vi "Simple App.vi"() -> ()   [LabVIEW 2014, in "SR3XXX HVPS.lvclass"]
uses:
  SR3XXX HVPS.lvclass
  reusable/Session APIs/Serial/Serial Session.lvclass
  reusable/Session APIs/Serial/Typedefs/Session Handle.ctl
panel:
  out "STB":bool[](array[boolean])
  out "ESB":bool[](array[boolean])
  in  "Power":bool
  out "voltage":dbl
  in  "Voltage Lim":dbl
  in  "Voltage SP":dbl
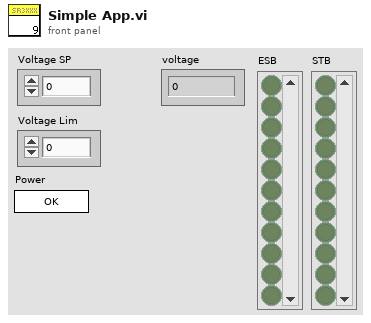
[diagram p1: front panel]
types:
  T1 = typedef "Serial Session.lvclass/Session Handle.ctl" = refnum<data-value>
  T2 = typedef "Session - Root.lvclass/Session Handle.ctl" = refnum<data-value>
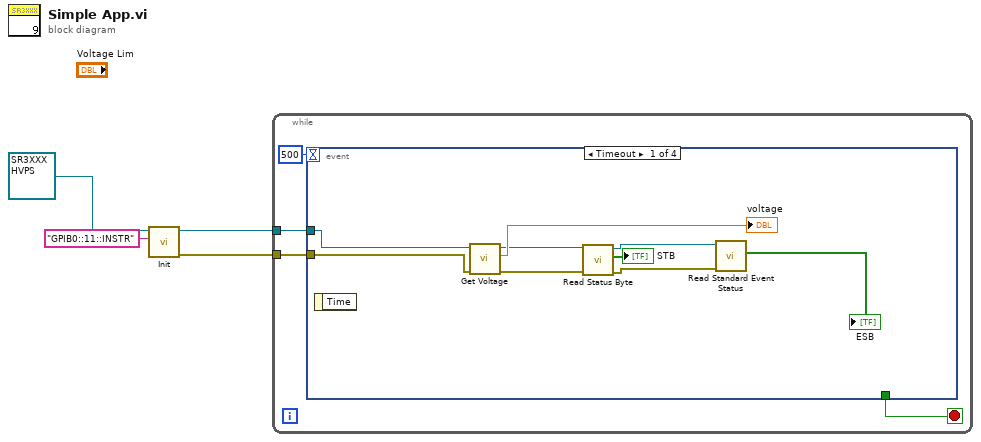
[diagram p0: block diagram]
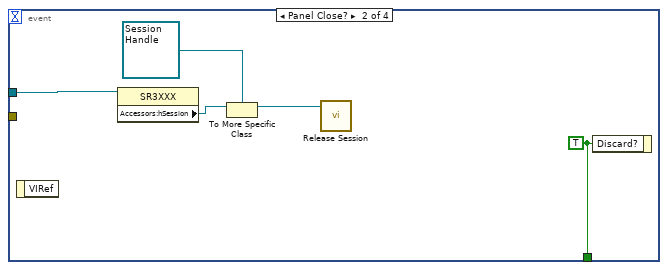
[diagram p2: hidden frame]
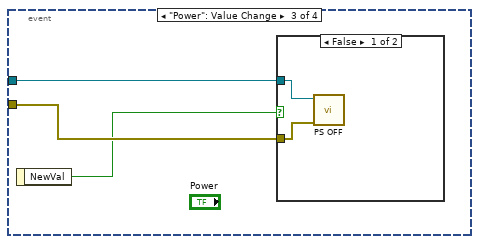
[diagram p3: hidden frame]
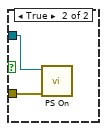
[diagram p4: hidden frame]
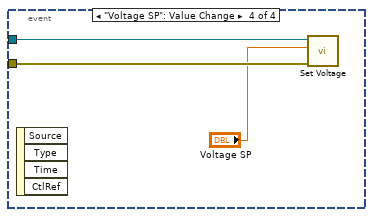
[diagram p5: hidden frame]
diagram:
  n1 = call-dynamic "Init.vi"("Session"="GPIB0::11::INSTR", "SR3XXX HVPS in"=refnum<class "SR3XXX HVPS.lvclass"> refnum) -> ("error out"=w1:errorcluster, "SR3XXX HVPS out"=w2:refnum<class "SR3XXX HVPS.lvclass">)  [unwired: 8 in]
  n2 = while {
    tunnel: w2 -> [w7]
    tunnel: w1 -> [w6]
    stop <- w8 stop-if-true
    n3 = event shown="[0] Timeout" {
      selector: _ -> [_ _ _ _]
      dyn-events: _ -> [_ _ _ _]
      timeout: 500 -> [_ _ _ _]
      tunnel: [_ w22 _ _] -> w8
      tunnel: w7 -> [w17 w21 w25 w32]
      tunnel: w6 -> [w16 _ w24 w31]
      event Timeout {
        n4 = event-data() -> ()  [unwired: 1 in, 1 out]
        n5 = call-dynamic "Get Voltage.vi"("error in (no error)"=w16, "SR3XXX HVPS in"=w17) -> ("error out"=w13:errorcluster, "V"=→"voltage":dbl, "SR3XXX HVPS out"=w14:refnum<class "SR3XXX HVPS.lvclass">)  [unwired: 7 in]
        n6 = call-dynamic "Read Status Byte.vi"("error in (no error)"=w13, "SR3XXX HVPS in"=w14) -> ("error out"=w11:errorcluster, "Byte"=→"STB":bool[], "SR3XXX HVPS out"=w12:refnum<class "SR3XXX HVPS.lvclass">)  [unwired: 7 in]
        n7 = call-dynamic "Read Standard Event Status.vi"("error in (no error)"=w11, "SR3XXX HVPS in"=w12) -> ("Byte"=→"ESB":bool[])  [unwired: 7 in, 2 out]
      }
      event Panel Close? {
        w22 = TRUE ("Discard?")
        n8 = event-data() -> ()  [unwired: 1 in, 1 out]
        n9 = property class="SR3XXX"(reference=w21) -> ("Accessors:hSession"=w20:T2)  [unwired: 1 in, 2 out]
        n10 = To More Specific Class(target class=T1 refnum ("Session Handle"), reference=w20) -> (specific class reference=w18:T1)  [unwired: 1 in, 1 out]
        n11 = call "Release Session.vi"("Session Handle"=w18) -> ()  [unwired: 14 in, 1 out]
        n12 = event-data("Discard?"=w22) -> ()  [unwired: 1 in, 1 out]
      }
      event "Power": Value Change {
        n13 = event-data() -> ("NewVal"=w23:bool)  [unwired: 1 in]
        n14 = case shown="False" w23 {
          tunnel: w25 -> [w27 w29]
          tunnel: w24 -> [w26 w28]
          frame False {
            n15 = call "PS OFF.vi"("error in"=w26, "SR3XXX in"=w27) -> ()  [unwired: 8 in, 2 out]
          }
          frame True {
            n16 = call "PS On.vi"("error in"=w28, "SR3XXX in"=w29) -> ()  [unwired: 8 in, 2 out]
          }
        }
      }
      event "Voltage SP": Value Change {
        n17 = event-data() -> ()  [unwired: 1 in, 4 out]
        n18 = call-dynamic "Set Voltage.vi"("error in (no error)"=w31, "V"="Voltage SP", "SR3XXX HVPS in"=w32) -> ()  [unwired: 7 in, 2 out]
      }
    }
  }
